vi "PH_GUI_Class.destructor.vi"(0 "i ref in":refnum<vi>, 5 "error in(no error)":errorcluster) -> (19 "error out":errorcluster)   [LabVIEW 2014, in "PH_GUI_Class.lvlib"]
doc: "This is the destructor of a class.\n\nLicense Agreement for this software:\n\nCopyright (C)\nGesellschaft für Schwerionenforschung, GSI\nPlanckstr. 1\n64291 Darmstadt\nGermany\n\nContact: D.Beck@gsi.de \n\nThis program is free software; you can redistribute it and/or modify it under the terms of the \nGNU General Public License as published by the Free Software Foundation; either version 2 of \nthe license, or (at your option) any later version.\n\nThis program is distributed in the hope that it will be useful, but WITHOUT ANY WARRANTY; \nwithout even the implied warranty of MERCHANTABILITY or FITNESS FOR A PARTICULAR PURPOSE. See the GNU General License for more details (http://www.gnu.org).\n\nGesellschaft für Schwerionenforschung, GSI\nPlanckstr. 1, 64291 Darmstadt, Germany\nFor all questions and ideas contact: M.Richter@gsi.de, H.Brand@gsi.de or D.Beck@gsi.de.\nLast update: 16-JUN-2004"
uses:
  PH_GUI_Class.lvlib
  CS_Core/BaseGUI/BaseGUI.lvlib
  PH_Common/PH_Common.lvlib
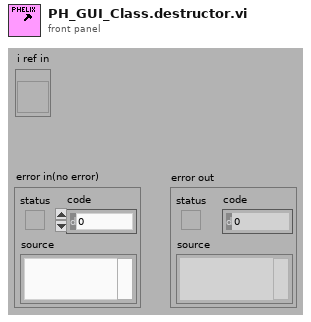
[diagram p1: front panel]
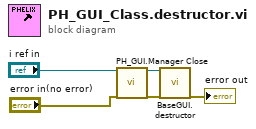
[diagram p0: block diagram]
diagram:
  n1 = call "PH_GUI.Manager Close.vi"("i ref in"="i ref in", "error in"="error in(no error)") -> ("i ref out"=w4:refnum<vi>, "error out"=w5:errorcluster)  [unwired: 16 in]
  n2 = call "BaseGUI.destructor.vi"("i ref in"=w4, "error in (no error)"=w5) -> ("error out"=→"error out":errorcluster)  [unwired: 17 in]
